vi "Identify XML Descriptor.vi"(8 "error in":errorcluster, 11 "XML Path in":path) -> (0 "error out":errorcluster, 2 "Found ?":bool, 3 "XML Path out":path, 5 "Custom Device Name":string, 7 "Common Doc Dir":string)   [LabVIEW 2019, in "LVLIBP CD XML Updater.lvlib" / "Project XML Editor.lvclass"]
uses:
  Project XML Editor.lvclass
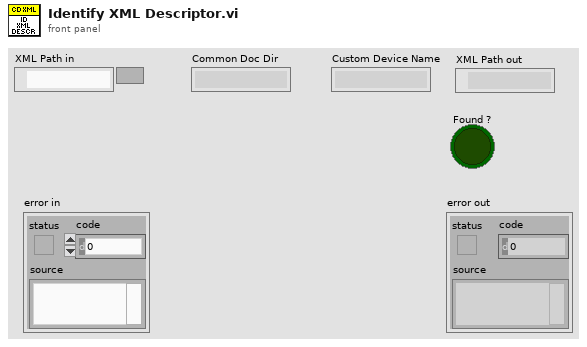
[diagram p1: front panel]
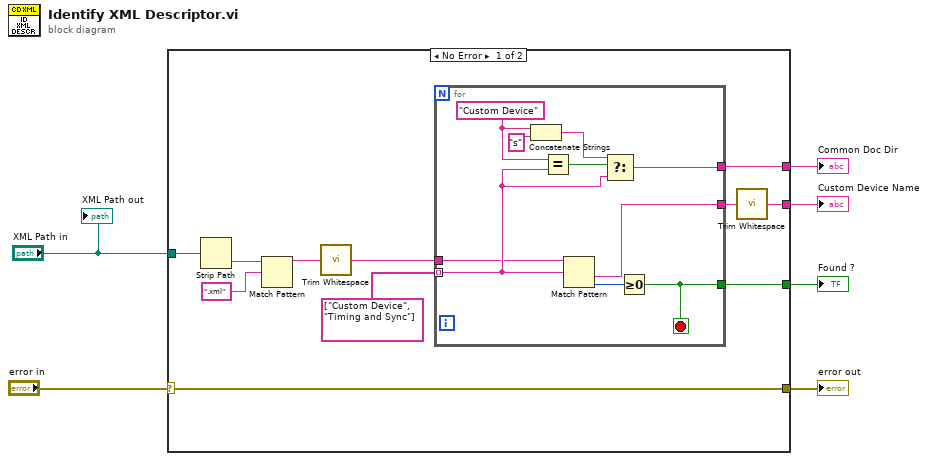
[diagram p0: block diagram]
diagram:
  n1 = case shown="No Error" "error in" {
    selector: "error in" -> [w9 w28]
    tunnel: "XML Path in" -> [w13 _]
    tunnel: [w9 w28] -> w5
    tunnel: [w7 _] -> w4
    tunnel: [w12 _] -> w3
    tunnel: [w10 _] -> w1
    frame No Error {
      n2 = Strip Path(path=w13) -> (name=w11:string)  [unwired: 1 out]
      n3 = Match Pattern(string=w11, regular expression=".xml") -> (before substring=w16:string)  [unwired: 1 in, 3 out]
      n4 = call <vilib>:"Trim Whitespace.vi"("string"=w16) -> ("trimmed string"=w17:string)  [unwired: 1 in]
      n5 = for {
        tunnel: string[] ["Custom Device", "Timing and Sync"] -> [w22] mode=indexing
        tunnel: w17 -> [w19]
        tunnel: [w18] -> w8
        tunnel: [w23] -> w12
        tunnel: [w20] -> w10
        stop <- w20 stop-if-true
        w26 = "Custom Device" ("y")
        n6 = Concatenate Strings(w26, "s" ("string")) -> (w24:string)
        n7 = Equal?(x=w26, y=w22) -> (x = y?=w27:bool)
        n8 = Match Pattern(string=w19, regular expression=w22) -> (after substring=w18:string, offset past match=w21:i32)  [unwired: 1 in, 2 out]
        n9 = Select(t=w24, s=w27, f=w22) -> (s? t:f=w23:string)
        n10 = Greater Or Equal To 0?(x=w21) -> (x >= 0?=w20:bool)
      }
      n11 = call <vilib>:"Trim Whitespace.vi"("string"=w8) -> ("trimmed string"=w7:string)  [unwired: 1 in]
    }
    frame Error {
    }
  }
  "error out" <- w5
  "Found ?" <- w1
  "Custom Device Name" <- w4
  "Common Doc Dir" <- w3
  "XML Path out" <- "XML Path in"
